vi "Load Script.vi"(5 "Script":string="beeper.beep(0.5,400)\ndelay(0.5)\nbeeper.beep(0.5, 800)\ndelay(0.5)\nbeeper.beep(0.5, 1200)", 7 "Script Name":string="myscript", 8 "error in":errorcluster, 9 "Save (No)":bool, 10 "Load Options (Load)":enum16{"Load", "Load & Run"}(ring), 11 "VISA resource name":refnum<visa-resource-name>) -> (0 "error out":errorcluster, 3 "VISA resource name out":refnum<visa-resource-name>, 4 "Command String":string)   [LabVIEW 2009, in "Keithley 2600 Series.lvlib"]
doc: "This VI will load a user script on to the instrument.\n\n<b>Note:</b> Scripts that are not syntactically correct may cause this VI to not execute properly. Please check your scripts with Test Script Builder before using them with this VI.\n\n<b>Functions and Attributes Used</b>\nloadscript <scriptname>\nendscript\n<scriptname>.save()\n<scriptname>.run()"
uses:
  <instrlib>/Keithley 2600 Series/Keithley 2600 Series.lvlib
panel:
  # "(c) 2008 Keithley Instruments, Inc.  ALL RIGHTS RESERVED."
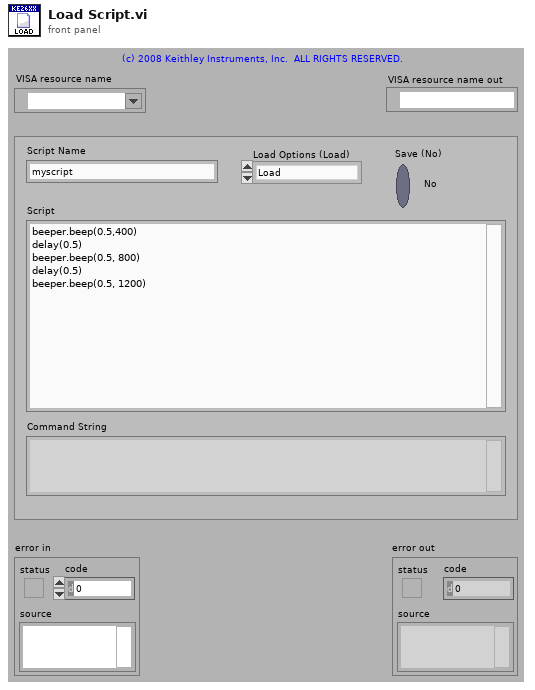
[diagram p1: front panel]
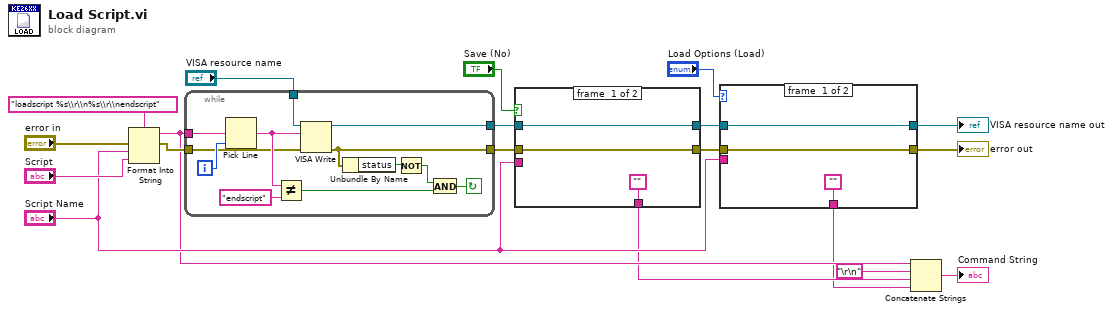
[diagram p0: block diagram]
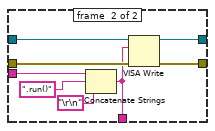
[diagram p2: hidden frame]
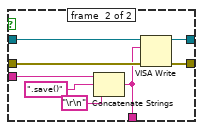
[diagram p3: hidden frame]
diagram:
  n1 = Format Into String(format string="loadscript %s\\r\\n%s\\r\\nendscript", error in="error in", "Script Name", "Script") -> (resulting string=w7:string, error out=w16:errorcluster)  [unwired: 1 in]
  n2 = while {
    tunnel: "VISA resource name" -> [w28]
    tunnel: w16 -> [w27]
    tunnel: [w24] -> w13
    tunnel: [w26] -> w12
    tunnel: w7 -> [w25]
    i -> [w30]
    stop <- w23 continue-if-true
    n3 = Pick Line(multi-line string=w25, line index=w30) -> (output string=w29:string)  [unwired: 1 out]
    n4 = Not Equal?(x=w29, y="endscript") -> (x != y?=w20:bool)
    n5 = VISA Write(VISA resource name=w28, write buffer=w29, error in (no error)=w27) -> (VISA resource name out=w26:refnum<visa-resource-name>, error out=w24:errorcluster)  [unwired: 1 out]
    n6 = Unbundle By Name(w24) -> ("status"=w22:bool)
    n7 = Not(x=w22) -> (.not. x?=w21:bool)
    n8 = And(x=w21, y=w20) -> (x .and. y?=w23:bool)
  }
  n9 = case shown="True" "Save (No)" {
    tunnel: w13 -> [w33 w41]
    tunnel: w12 -> [w34 w42]
    tunnel: "Script Name" -> [_ w39]
    tunnel: [w34 w38] -> w10
    tunnel: [w33 w37] -> w9
    tunnel: ["" w36] -> w4
    frame #0 {
    }
    frame #1 {
      n10 = Concatenate Strings(w39, ".save()" ("string"), "\r\n") -> (w36:string)
      n11 = VISA Write(VISA resource name=w42, write buffer=w36, error in (no error)=w41) -> (VISA resource name out=w38:refnum<visa-resource-name>, error out=w37:errorcluster)  [unwired: 1 out]
    }
  }
  n12 = case shown="\"Load & Run\"" "Load Options (Load)" {
    tunnel: w10 -> [w45 w53]
    tunnel: w9 -> [w44 w52]
    tunnel: "Script Name" -> [_ w50]
    tunnel: [w45 w49] -> w2
    tunnel: [w44 w48] -> w1
    tunnel: ["" w47] -> w3
    frame #0 {
    }
    frame #1 {
      n13 = Concatenate Strings(w50, ".run()" ("string"), "\r\n") -> (w47:string)
      n14 = VISA Write(VISA resource name=w53, write buffer=w47, error in (no error)=w52) -> (VISA resource name out=w49:refnum<visa-resource-name>, error out=w48:errorcluster)  [unwired: 1 out]
    }
  }
  "error out" <- w1
  "VISA resource name out" <- w2
  n15 = Concatenate Strings(w7, "\r\n", w4, w3) -> (→"Command String":string)
